vi "SVN_ParseTimeStamp.vi"(11 "Timestring (In)":string="2018-04-07T20:16:29,107705Z") -> (3 "Timestamp (Out)":timestamp)   [LabVIEW 2014]
panel:
  out "error out":errorcluster
  # "convert SVN-ISO 8601-timestring to Timestamp (not abs.)"
  # "the VI is reentrant"
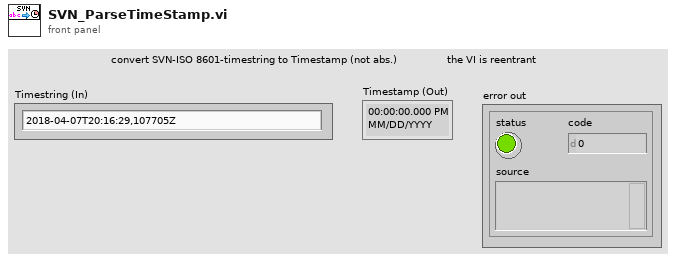
[diagram p1: front panel]
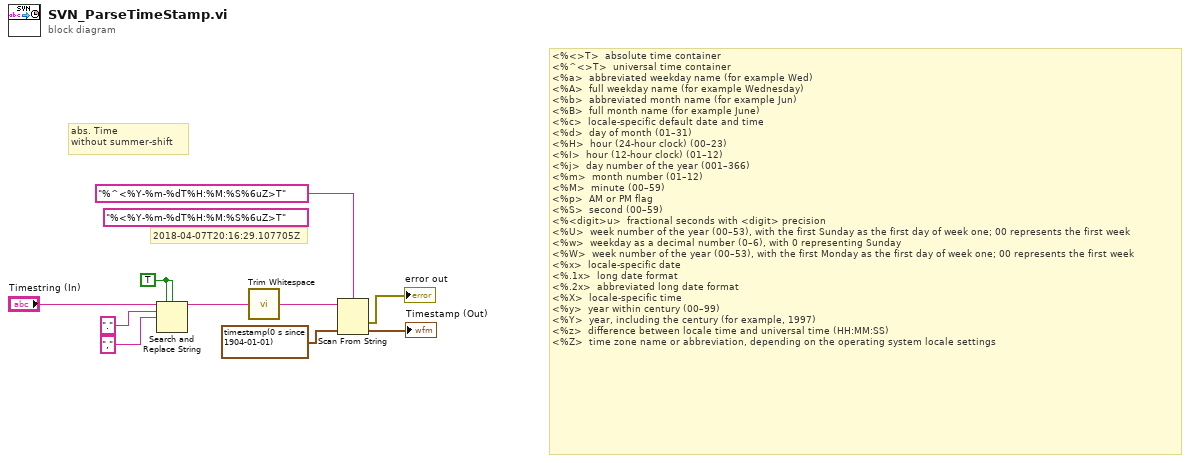
[diagram p0: block diagram]
diagram:
  w4 = TRUE ("replace all? (F)")
  (unwired) "%<%Y-%m-%dT%H:%M:%S%6uZ>T" ("format string")
  # "2018-04-07T20:16:29.107705Z"
  # "abs. Time\nwithout summer-shift"
  # "<%<>T> \tabsolute time container\n<%^<>T> \tuniversal time container\n<%a> \tabbreviated weekday name (for example Wed)\n<%A> \tfull weekday name (for example Wednesday)\n<%b> \tabbreviated month name (for example Jun)\n<%B> \tfull month name (for example June)\n<%c> \tlocale-specific default date and time\n<%d> \tday of month (01–31)\n<%H> \thour (24-hour clock) (00–23)\n<%I> \thour (12-hour clock) (01–12)\n<%j> \tday number of the year (001–366)\n<%m> \tmonth number (01–12)\n<%M> \tminute (00–59)\n<%p> \tAM or PM flag\n<%S> \tsecond (00–59)\n<%<digit>u> \tfractional seconds with <digit> precision\n<%U> \tweek number of the year (00–53), with the first Sunday as the first day of week one; 00 represents the first week\n<%w> \tweekday as a decimal number (0–6), with 0 representing Sunday\n<%W> \tweek number of the year (00–53), with the first Monday as the first day of week one; 00 represents the first week\n<%x> \tlocale-specific date\n<%.1x> \tlong date format\n<%.2x> \tabbreviated long date format\n<%X> \tlocale-specific time\n<%y> \tyear within century (00–99)\n<%Y> \tyear, including the century (for example, 1997)\n<%z> \tdifference between locale time and universal time (HH:MM:SS)\n<%Z> \ttime zone name or abbreviation, depending on the operating system locale settings"
  n1 = Search and Replace String(replace all?=w4, case sensitive?=w4, input string="Timestring (In)", search string=".", replace string="," ("replace string (\"\")")) -> (result string=w3:string)  [unwired: 3 in, 3 out]
  n2 = call <vilib>:"Trim Whitespace.vi"("string"=w3) -> ("trimmed string"=w8:string)  [unwired: 1 in]
  n3 = Scan From String(format string="%^<%Y-%m-%dT%H:%M:%S%6uZ>T", input string=w8, default 1=timestamp(0 s since 1904-01-01) ("Time Stamp")) -> (error out=→"error out":errorcluster, output 1=→"Timestamp (Out)":timestamp)  [unwired: 2 in, 2 out]
